vi "Begin.vi"() -> (0 "error out":errorcluster)   [LabVIEW 2013]
doc: "Called before other user functions, this VI is expected to open initial I/O refnums, load in file data, and do all program initialization. Notice that the <B>error out</B> terminal is simply used for data flow. Wiring it to other structures or subVIs ensures that this VI runs first."
uses:
  <vilib>/Rock Robotics/WPI/DriverStation/WPI_DriverStationRobotMode2.ctl
  <vilib>/Rock Robotics/SystemInterfaces/DIO/FPGA_DIOChannel.ctl
  Robot Global Data.vi
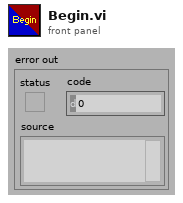
[diagram p1: front panel]
types:
  T1 = typedef "FPGA_DIOChannel.ctl" = enum8{"DIO 1", "DIO 2", "DIO 3", "DIO 4", "DIO 5", "DIO 6", "DIO 7", "DIO 8", "DIO 9", "DIO 10", "DIO 11", "DIO 12", "DIO 13", "DIO 14", "Invalid"}
  T2 = typedef "WPI_DriverStationRobotMode2.ctl" = enum16{"Autonomous Disabled", "Autonomous Enabled", "Teleop Disabled", "Teleop Enabled", "Timeout", "Finish", "Test Disabled", "Test Enabled"}
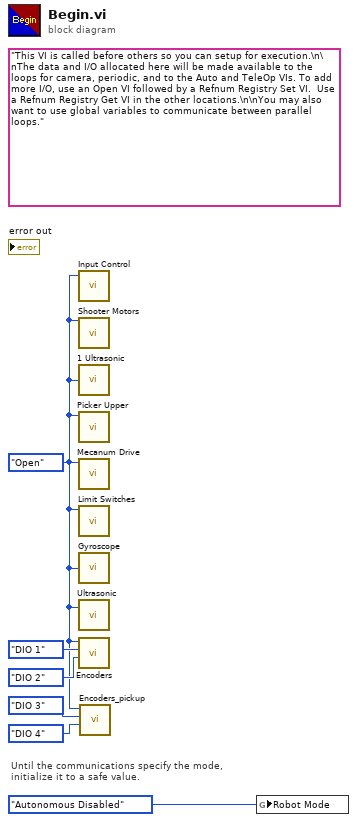
[diagram p0: block diagram]
diagram:
  w3 = enum16{"Open", "Run", "End"}."Open" ("State Control")
  (unwired) "This VI is called before others so you can setup for execution.\n\nThe data and I/O allocated here will be made available to the loops for camera, periodic, and to the Auto and TeleOp VIs. To add more I/O, use an Open VI followed by a Refnum Registry Set VI.  Use a Refnum Registry Get VI in the other locations.\n\nYou may also want to use global variables to communicate between parallel loops."
  # "Until the communications specify the mode,\ninitialize it to a safe value."
  n1 = call "Input Control.vi"("State"=w3) -> ()  [unwired: 2 in, 3 out]
  n2 = call "Shooter Motors.vi"("State Control"=w3) -> ()  [unwired: 16 in, 3 out]
  n3 = call "1 Ultrasonic.vi"("State Control"=w3) -> ()  [unwired: 1 out]
  n4 = call "Picker Upper.vi"("State Control"=w3) -> ()  [unwired: 10 in, 1 out]
  n5 = call "Mecanum Drive.vi"("State Control"=w3) -> ()  [unwired: 7 in]
  n6 = call "Limit Switches.vi"("State Control"=w3) -> ()  [unwired: 7 in, 4 out]
  n7 = call "Gyroscope.vi"("State Control"=w3) -> ()  [unwired: 2 out]
  n8 = call "Ultrasonic.vi"("State Control"=w3) -> ()  [unwired: 2 in]
  n9 = call "Encoders.vi"("B Channel"=FPGA_DIOChannel."DIO 2", "A Channel"=FPGA_DIOChannel."DIO 1", "State Control"=w3) -> ()  [unwired: 1 in, 4 out]
  n10 = call "Encoders_pickup.vi"("B Channel"=FPGA_DIOChannel."DIO 4", "A Channel"=FPGA_DIOChannel."DIO 3", "State Control"=w3) -> ()  [unwired: 1 in, 4 out]
  n11 = global write "Robot Global Data.vi" "Robot Mode"(WPI_DriverStationRobotMode2."Autonomous Disabled" ("Robot Mode")) -> ()
